vi "Fetch Single Record Multiple Channel.vi"   [LabVIEW 2011]
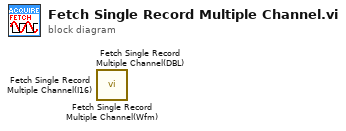
[diagram p0: block diagram]
diagram:
  n1 = call <userlib>:"Fetch Single Record Multiple Channel(Wfm).vi"() -> ()  [unwired: 9 in, 3 out]
  n2 = call <userlib>:"Fetch Single Record Multiple Channel(DBL).vi"() -> ()  [unwired: 9 in, 3 out]
  n3 = call <userlib>:"Fetch Single Record Multiple Channel(I16).vi"() -> ()  [unwired: 9 in, 3 out]
